vi "Fill Text.vi"(7 "String ref":refnum<vi>, 10 "Error In":errorcluster, 11 "String in":string) -> (2 "Error Out":errorcluster)   [LabVIEW 2019, in "Tools.lvlib"]
uses:
  Tools.lvlib
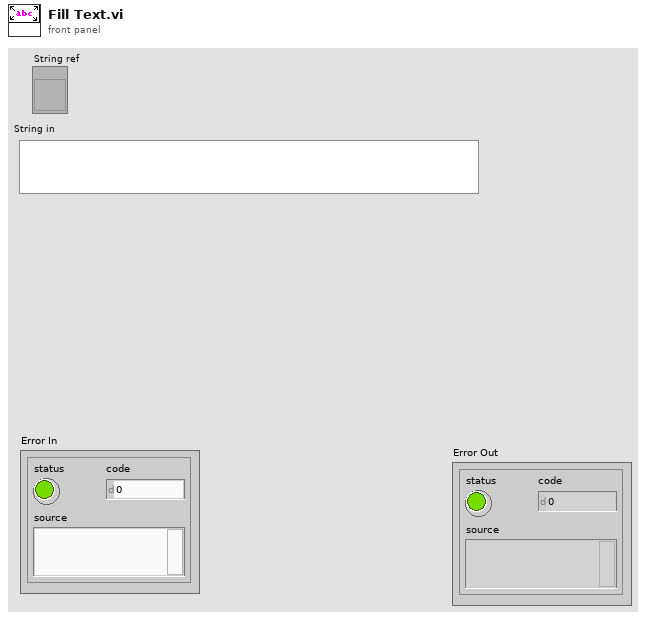
[diagram p1: front panel]
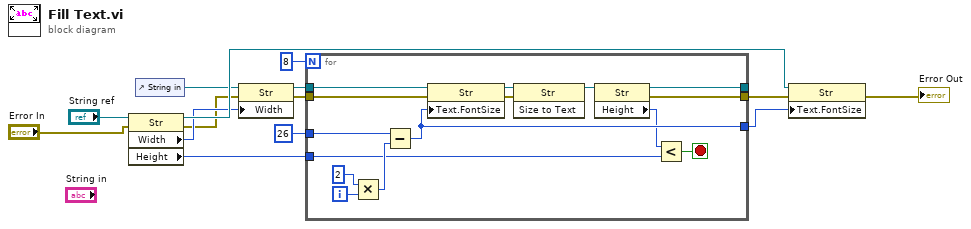
[diagram p0: block diagram]
diagram:
  n1 = property class="Str"(reference="String ref", error in="Error In") -> (reference out=w8:refnum<vi>, error out=w1:errorcluster, "Width"=w6:u32, "Height"=w13:u32)
  n2 = control-ref of="String in"() -> (w7:refnum<vi>)
  n3 = property class="Str"(reference=w7, error in=w1, "Width"=w6) -> (reference out=w5:refnum<vi>, error out=w4:errorcluster)
  n4 = for {
    N: 8 -> [_]
    tunnel: i16 26 ("Size") -> [w29]
    tunnel: w5 -> [w25]
    tunnel: w13 -> [w17]
    tunnel: [w22] -> w11
    tunnel: [w21] -> _
    tunnel: [w16] -> w9
    tunnel: w4 -> [w15]
    i -> [w28]
    stop <- w23 stop-if-true
    n5 = Multiply(x=2, y=w28) -> (x*y=w20:i32)
    n6 = Subtract(x=w29, y=w20) -> (x-y=w22:i32)
    n7 = property class="Str"(reference=w25, error in=w15, "Text.FontSize"=w22) -> (reference out=w26:refnum<vi>, error out=w27:errorcluster)
    n8 = invoke class="Str" method="Size to Text"(reference=w26, error in=w27) -> (reference out=w24:refnum<vi>)  [unwired: 1 in, 2 out]
    n9 = property class="Str"(reference=w24) -> (reference out=w21:refnum<vi>, error out=w16:errorcluster, "Height"=w18:u32)  [unwired: 1 in]
    n10 = Less?(x=w18, y=w17) -> (x < y?=w23:bool)
  }
  n11 = property class="Str"(reference=w8, error in=w9, "Text.FontSize"=w11) -> (error out=→"Error Out":errorcluster)  [unwired: 1 out]
